vi "Close Reference.vi"(0 "LV Doc in":refnum<class "LV Doc.lvclass">, 11 "error in (no error)":errorcluster) -> (4 "LV Doc out":refnum<class "LV Doc.lvclass">, 15 "error out":errorcluster)   [LabVIEW 2016, in "LV Doc.lvclass"]
uses:
  LV Doc.lvclass
  D:/MDI Project/source code/Document/Document.lvclass
  Document.lvclass/Document.ctl
  LV Doc.lvclass/LV Doc.ctl
  Document.lvclass
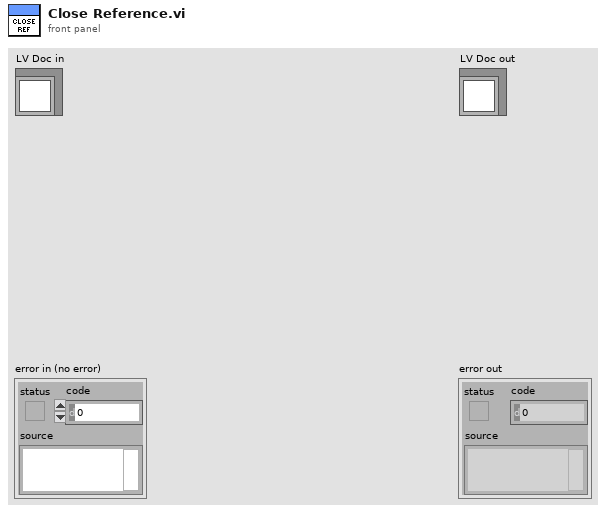
[diagram p1: front panel]
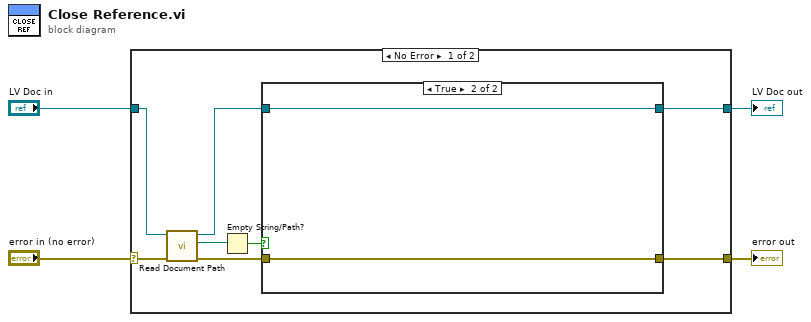
[diagram p0: block diagram]
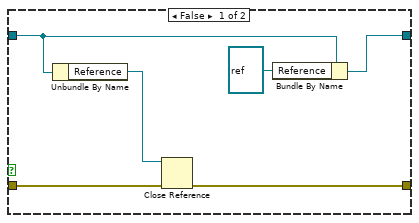
[diagram p2: hidden frame]
diagram:
  n1 = case shown="No Error" "error in (no error)" {
    selector: "error in (no error)" -> [w8 w22]
    tunnel: [w12 w22] -> w3
    tunnel: [w11 w21] -> w1
    tunnel: "LV Doc in" -> [w10 w21]
    frame No Error {
      n2 = call "Read Document Path.vi"("error in (no error)"=w8, "Document in"=w10) -> ("error out"=w7:errorcluster, "Document Path"=w6:path, "Document out"=w9:refnum<class "LV Doc.lvclass">)  [unwired: 7 in]
      n3 = Empty String/Path?(string/path=w6) -> (empty?=w5:bool)
      n4 = case shown="True" w5 {
        tunnel: [w18 w19] -> w12
        tunnel: [w16 w20] -> w11
        tunnel: w9 -> [w14 w20]
        tunnel: w7 -> [w13 w19]
        frame False {
          n5 = Unbundle By Name(w14) -> ("Reference"=w17:refnum<vi>)
          n6 = Close Reference(reference=w17, error in (no error)=w13) -> (error out=w18:errorcluster)
          n7 = Bundle By Name(cluster=w14, "Reference"=refnum<vi> refnum) -> (w16:refnum<class "LV Doc.lvclass">)
        }
        frame True {
        }
      }
    }
    frame Error {
    }
  }
  "error out" <- w3
  "LV Doc out" <- w1
